vi "Configure Function.vi"(8 "error in (no error)":errorcluster, 10 "Function (Sine)":T1(ring), 11 "VISA resource name":refnum<visa-resource-name>) -> (0 "error out":errorcluster, 3 "VISA resource name out":refnum<visa-resource-name>)   [LabVIEW 2017, in "Keithley 3390.lvlib"]
doc: "Sets the output waveform function."
uses:
  Keithley 3390.lvlib
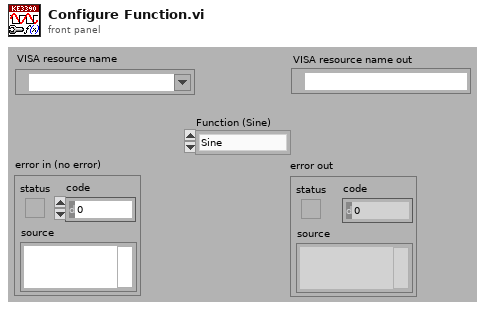
[diagram p1: front panel]
types:
  T1 = enum16{"Sine", "Square", "Ramp", "Pulse", "Noise", "DC", "Arbitrary"}
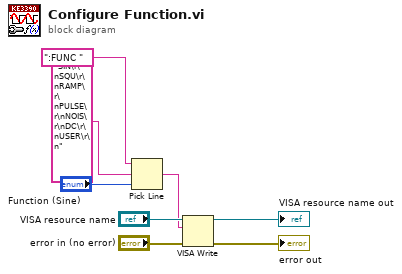
[diagram p0: block diagram]
diagram:
  n1 = Pick Line(string ("")=":FUNC " ("command"), multi-line string="SIN\r\nSQU\r\nRAMP\r\nPULSE\r\nNOIS\r\nDC\r\nUSER\r\n" ("options"), line index="Function (Sine)") -> (output string=w3:string)
  n2 = VISA Write(VISA resource name="VISA resource name", write buffer=w3, error in (no error)="error in (no error)") -> (VISA resource name out=→"VISA resource name out":refnum<visa-resource-name>, error out=→"error out":errorcluster)  [unwired: 1 out]
